vi "brutal_stop.vi"(0 "Button Reference":refnum<vi>) -> ()   [LabVIEW 2010]
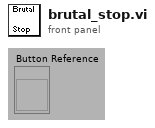
[diagram p1: front panel]
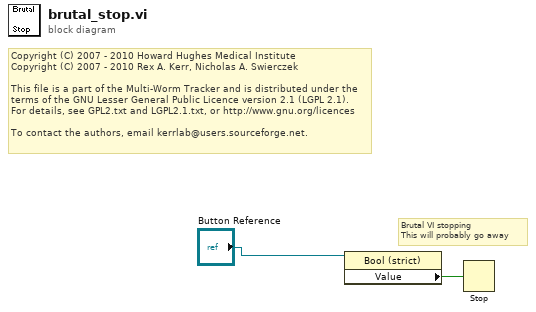
[diagram p0: block diagram]
diagram:
  # "Copyright (C) 2007 - 2010 Howard Hughes Medical Institute\nCopyright (C) 2007 - 2010 Rex A. Kerr, Nicholas A. Swierczek\n \nThis file is a part of the Multi-Worm Tracker and is distributed under the\nterms of the GNU Lesser General Public Licence version 2.1 (LGPL 2.1).\nFor details, see GPL2.txt and LGPL2.1.txt, or http://www.gnu.org/licences\n \nTo contact the authors, email kerrlab@users.sourceforge.net."
  # "Brutal VI stopping\nThis will probably go away"
  n1 = property class="Bool (strict)"(reference="Button Reference") -> ("Value"=w2:bool)  [unwired: 1 in, 2 out]
  n2 = Stop(stop? (T)=w2) -> ()
